vi "Trim Whitespace.vi"(0 "string":string, 1 "location (both)":T1 items=["both", "start of string", "end of string"]) -> (2 "trimmed string":string)   [LabVIEW 2022 SP3]
doc: "Removes all ASCII white space (spaces, tabs, carriage returns, and linefeeds) from the beginning, end, or both ends of <B>string</B>. The Trim Whitespace VI does not remove double byte characters."
uses:
  whitespace.ctl
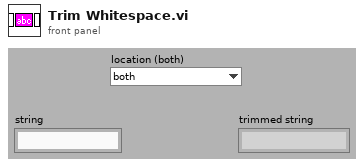
[diagram p1: front panel]
types:
  T1 = typedef "whitespace.ctl" = u16
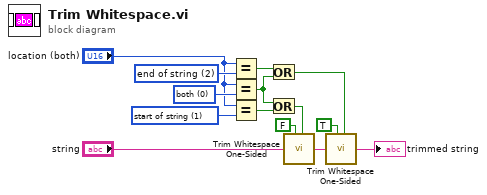
[diagram p0: block diagram]
diagram:
  w7 = T1 2 items=["both", "start of string", "end of string"] ("y")
  w12 = T1 1 items=["both", "start of string", "end of string"] ("y")
  w13 = T1 0 items=["both", "start of string", "end of string"] ("y")
  n1 = Equal?(x="location (both)", y=w7) -> (x = y?=w4:bool)
  n2 = Equal?(x="location (both)", y=w13) -> (x = y?=w5:bool)
  n3 = Equal?(x="location (both)", y=w12) -> (x = y?=w10:bool)
  n4 = Or(x=w4, y=w5) -> (x .or. y?=w6:bool)
  n5 = Or(x=w5, y=w10) -> (x .or. y?=w11:bool)
  n6 = call "Trim Whitespace One-Sided.vi"("string"="string", "reverse?"=FALSE, "enable?"=w11) -> ("trimmed string"=w9:string)
  n7 = call "Trim Whitespace One-Sided.vi"("string"=w9, "reverse?"=TRUE, "enable?"=w6) -> ("trimmed string"=→"trimmed string":string)
